vi "VNA De-embedding - SParam.vi"(8 "error in":errorcluster, 10 "RFmxVNA Settings":T1={"Resource Name"="", "vCal Name"="", "RFmxVNA Calset Enable"=FALSE, "RFmxVNA Calset Interpolation"=FALSE, "Calset File Path"="", "RFmxVNA attenuation mode"=enum."s2p File", "RFmxVNA Port1 s2p file path"="", "RFmxVNA Port1 s-parameters orientation"=enum."Port1 Towards DUT", "RFmxVNA Port1 Power Compensation"=FALSE, "RFmxVNA Port2 s2p file path"="", "RFmxVNA Port2 s-parameters orientation"=enum."Port1 Towards DUT", "RFmxVNA Port2 Power Compensation"=FALSE, "Port1 Power Level (dBm)"=0.0, "Port1 Test Receiver Attenuation (dB)"=0.0, "Port2 Power Level (dBm)"=0.0, "Port2 Test Receiver Attenuation (dB)"=0.0, "IF Bandwidth (Hz)"=0.0, "Frequency Sweep"={"Start Frequency (Hz)"=4000000000.0, "Stop Frequency (Hz)"=26000000000.0, "Number of Points"=200}} {"Frequency Sweep"."Stop Frequency (Hz)" format="%.3p"; "Frequency Sweep"."Start Frequency (Hz)" format="%.3p"; "IF Bandwidth (Hz)" format="%.2p"; "Port2 Test Receiver Attenuation (dB)" format="%.2f"; "Port2 Power Level (dBm)" format="%.2f"; "Port1 Test Receiver Attenuation (dB)" format="%.2f"; "Port1 Power Level (dBm)" format="%.2f"}, 11 "RFmxVNA Session in":refnum<k21>) -> (0 "error out":errorcluster, 3 "RFmxVNA Session out":refnum<k21>)   [LabVIEW 2023]
uses:
  Controls/RFmxVNA Config - SParam.ctl
  <vilib>/Utility/error.llb/Trim Whitespace.vi
  <vilib>/Utility/error.llb/Trim Whitespace One-Sided.vi
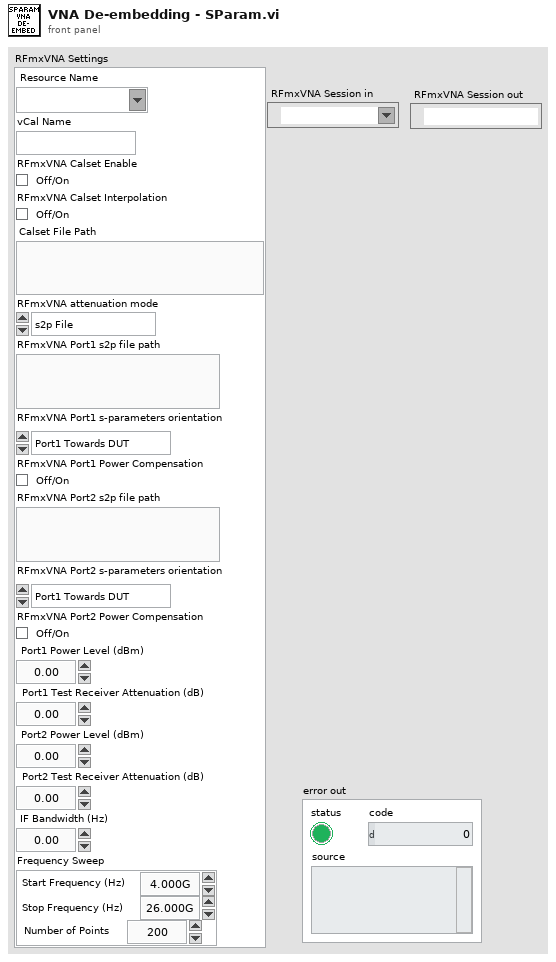
[diagram p1: front panel]
types:
  T1 = typedef "RFmxVNA Config - SParam.ctl" = cluster{"Resource Name":refnum<k15>, "vCal Name":string, "RFmxVNA Calset Enable":bool, "RFmxVNA Calset Interpolation":bool, "Calset File Path":string, "RFmxVNA attenuation mode":enum32{"<None>", "s2p File"}, "RFmxVNA Port1 s2p file path":string, "RFmxVNA Port1 s-parameters orientation":enum32{"Port1 Towards DUT", "Port2 Towards DUT"}, "RFmxVNA Port1 Power Compensation":bool, "RFmxVNA Port2 s2p file path":string, "RFmxVNA Port2 s-parameters orientation":enum32{"Port1 Towards DUT", "Port2 Towards DUT"}, "RFmxVNA Port2 Power Compensation":bool, "Port1 Power Level (dBm)":dbl, "Port1 Test Receiver Attenuation (dB)":dbl, "Port2 Power Level (dBm)":dbl, "Port2 Test Receiver Attenuation (dB)":dbl, "IF Bandwidth (Hz)":dbl, "Frequency Sweep":cluster{"Start Frequency (Hz)":dbl, "Stop Frequency (Hz)":dbl, "Number of Points":i32}}
  T2 = cluster{"Port Name":string, "S2P File Path":string, "S-parameter Orientation":i32, "Power Compensation Enabled":i32}
  T3 = cluster{"Port Name":string, "S2P File Path":string, "S-parameter Orientation":i32, "Power Compensation Enabled":i32}[]
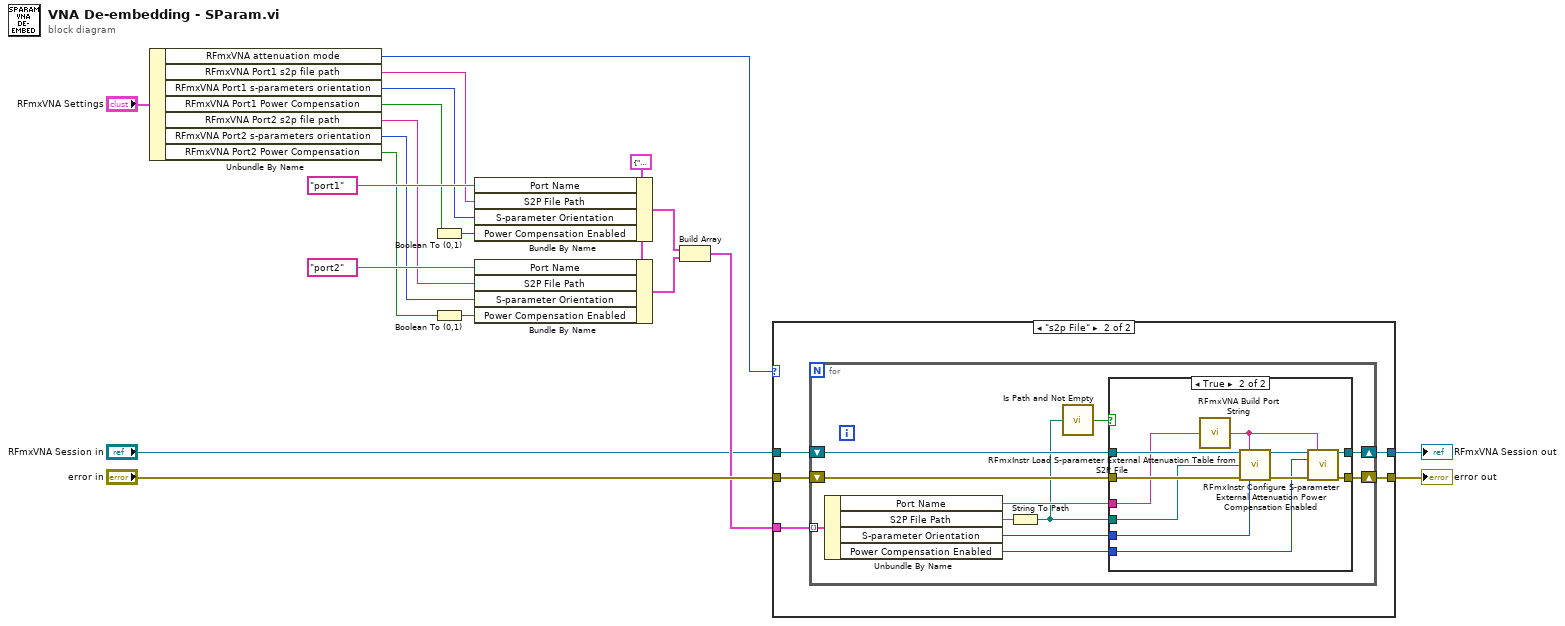
[diagram p0: block diagram]
diagram:
  w16 = T2 {"Port Name"="port1", "S2P File Path"="Support\\1dB_Attenuation.s2p", "S-parameter Orientation"=1, "Power Compensation Enabled"=1} ("Cluster")
  n1 = Unbundle By Name("RFmxVNA Settings") -> ("RFmxVNA attenuation mode"=w2:enum32{"<None>", "s2p File"}, "RFmxVNA Port1 s2p file path"=w13:string, "RFmxVNA Port1 s-parameters orientation"=w11:enum32{"Port1 Towards DUT", "Port2 Towards DUT"}, "RFmxVNA Port1 Power Compensation"=w5:bool, "RFmxVNA Port2 s2p file path"=w12:string, "RFmxVNA Port2 s-parameters orientation"=w10:enum32{"Port1 Towards DUT", "Port2 Towards DUT"}, "RFmxVNA Port2 Power Compensation"=w3:bool)
  n2 = Boolean To (0,1)(Boolean=w5) -> (0, 1=w6:i16)
  n3 = Boolean To (0,1)(Boolean=w3) -> (0, 1=w4:i16)
  n4 = Bundle By Name(cluster=w16, "Port Name"="port1" ("Port"), "S2P File Path"=w13, "S-parameter Orientation"=w11, "Power Compensation Enabled"=w6) -> (w9:T2)
  n5 = Bundle By Name(cluster=w16, "Port Name"="port2" ("Port"), "S2P File Path"=w12, "S-parameter Orientation"=w10, "Power Compensation Enabled"=w4) -> (w8:T2)
  n6 = Build Array(w9, w8) -> (w7:T3)
  n7 = case shown="\"s2p File\"" w2 {
    tunnel: "RFmxVNA Session in" -> [w22 w27]
    tunnel: "error in" -> [w21 w26]
    tunnel: [w22 w25] -> w18
    tunnel: [w21 w24] -> w17
    tunnel: w7 -> [_ w23]
    frame "<None>", Default {
    }
    frame "s2p File" {
      n8 = for {
        shift-right: [w32] -> w25
        shift-left: w27 -> [w38]
        shift-right: [w33] -> w24
        shift-left: w26 -> [w37]
        tunnel: w23 -> [w34] mode=indexing
        n9 = Unbundle By Name(w34) -> ("Port Name"=w36:string, "S2P File Path"=w29:string, "S-parameter Orientation"=w35:i32, "Power Compensation Enabled"=w31:i32)
        n10 = String To Path(string=w29) -> (path=w28:path)
        n11 = call <vilib>:"Is Path and Not Empty.vi"("path"=w28) -> ("Is Path and Not Empty?"=w30:bool)  [unwired: 4 in]
        n12 = case shown="True" w30 {
          tunnel: w38 -> [w40 w51]
          tunnel: w37 -> [w39 w50]
          tunnel: w36 -> [_ w48]
          tunnel: w35 -> [_ w47]
          tunnel: [w39 w46] -> w33
          tunnel: [w40 w44] -> w32
          tunnel: w31 -> [_ w43]
          tunnel: w28 -> [_ w41]
          frame False {
          }
          frame True {
            n13 = call <vilib>:"RFmxVNA Build Port String.vi"("Port Name"=w48) -> ("Selector String Out"=w42:string)  [unwired: 14 in]
            n14 = call <vilib>:"RFmxInstr Load S-parameter External Attenuation Table from S2P File.vi"("Instrument Handle In"=w51, "Selector String"=w42, "S2P File Path"=w41, "error in (no error)"=w50, "S-parameter Orientation"=w47) -> ("Instrument Handle Out"=w45:refnum<k21>, "error out"=w49:errorcluster)  [unwired: 9 in]
            n15 = call <vilib>:"RFmxInstr Configure S-parameter External Attenuation Power Compensation Enabled.vi"("Instrument Handle In"=w45, "Selector String"=w42, "Power Compensation Enabled"=w43, "error in (no error)"=w49) -> ("Instrument Handle Out"=w44:refnum<k21>, "error out"=w46:errorcluster)  [unwired: 10 in]
          }
        }
      }
    }
  }
  "error out" <- w17
  "RFmxVNA Session out" <- w18
